vi "test_SessionReservationInfo_ReserveSessions_SessionAnnotationsPopulated.vi"(8 "error in":errorcluster) -> (0 "error out":errorcluster, 2 "result":string, 3 "pass":bool)   [LabVIEW 2021, in "MeasurementServerTests.lvlib" / "Session Reservation Tests.lvlib"]
uses:
  Session Reservation Tests.lvlib
  gRPC/Generated APIs/ni/measurementlink/sessionmanagement/v1/RPC Messages/ni_measurementlink_PinMapContext.ctl
  Runtime/Clients/Session Management V1/Session Reservation/Session Reservation.lvclass/Session Reservation.ctl
  bff49ccc-0781-4f8a-a739-0c4a6493da00.vi
  c21ecf1c-8bb5-4f68-90ba-61375d462941.vi
  Runtime/Clients/Session Management V1/Session Reservation/Merge Invalid DVR Error.vi
  Helpers/Pin Map XML Strings Global.vi
  Runtime/Clients/Session Management V1/Session Reservation/Is DVR Valid.vi
  Runtime/Measurements/Helpers/Error Strings Global Internal.vi
  <vilib>/Utility/error.llb/Error Cluster From Error Code.vi
  <vilib>/JDP Science/JSONtext/Variant to JSON Text.vi
  <vilib>/JDP Science/JSONtext/LVClass Serializer/JSONtext LVClass Serializer.lvclass
  gRPC/Generated APIs/ni/measurementlink/sessionmanagement/v1/ni.measurementlink.sessionmanagement.v1.api.lvlib
  MeasurementServerTests.lvlib
  Runtime/Clients/Session Management V1/Session Reservation/Session Reservation.lvclass
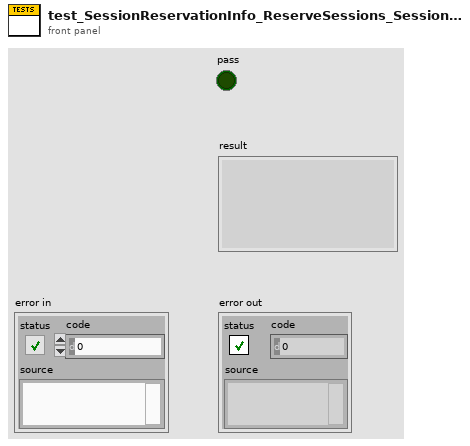
[diagram p1: front panel]
types:
  T1 = typedef "ni.measurementlink.sessionmanagement.v1.api.lvlib/ni_measurementlink_PinMapContext.ctl" = cluster{"pin_map_id":string, "sites":i32[]}
  T2 = typedef "ni.measurementlink.sessionmanagement.v1.api.lvlib/ni_measurementlink_sessionmanagement_v1_SessionInformation_AnnotationsEntry.ctl" = cluster{"key":string, "value":string}
  T3 = typedef "ni.measurementlink.sessionmanagement.v1.api.lvlib/ni_measurementlink_sessionmanagement_v1_SessionInformation.ctl" = cluster{"session":T4, "resource_name":string, "channel_list":string, "instrument_type_id":string, "session_exists":bool, "session_reserved":bool, "channel_mappings":T5[], "annotations":T2[]}
  T4 = typedef "ni.measurementlink.sessionmanagement.v1.api.lvlib/nidevice_grpc_Session.ctl" = cluster{"name":string}
  T5 = typedef "ni.measurementlink.sessionmanagement.v1.api.lvlib/ni_measurementlink_sessionmanagement_v1_ChannelMapping.ctl" = cluster{"pin_or_relay_name":string, "site":i32, "channel":string, "multiplexer_resource_name":string, "multiplexer_route":string}
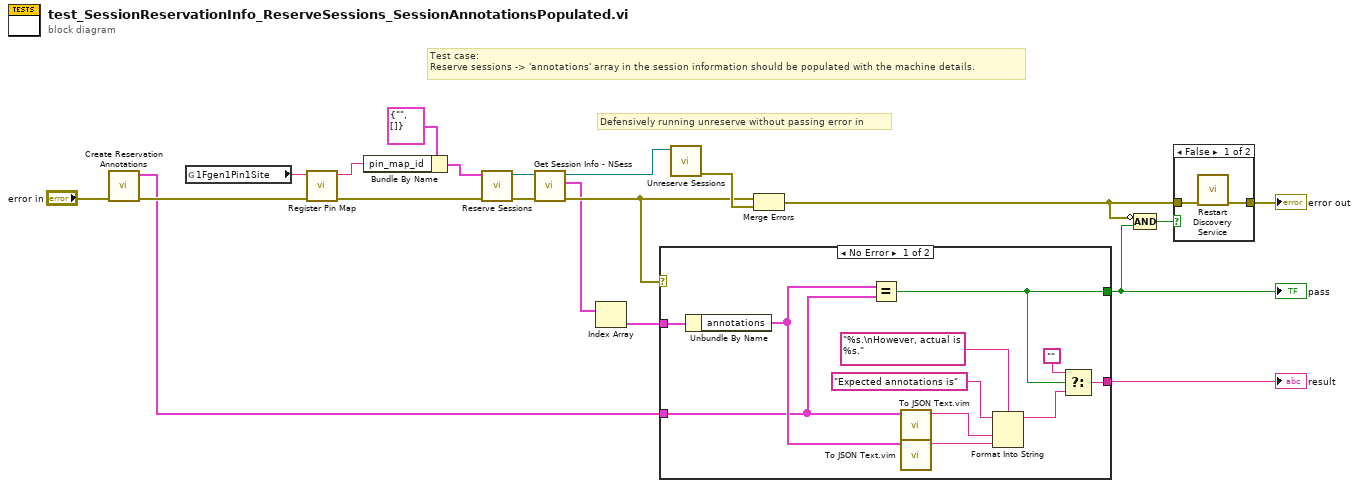
[diagram p0: block diagram]
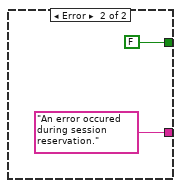
[diagram p3: hidden frame]
diagram:
  # "Defensively running unreserve without passing error in"
  # "Test case:\nReserve sessions -> 'annotations' array in the session information should be populated with the machine details."
  n1 = call "Create Reservation Annotations.vi"("error in"="error in") -> ("error out"=w10:errorcluster, "annotations array"=w6:T2[])  [unwired: 9 in]
  n2 = global read "Pin Map XML Strings Global.vi" "1Fgen1Pin1Site"() -> (w1:string)
  n3 = call "Register Pin Map.vi"("error in"=w10, "pin map xml"=w1) -> ("error out"=w16:errorcluster, "pin map id"=w17:string)  [unwired: 8 in]
  n4 = Bundle By Name(cluster=T1 {"pin_map_id"="", "sites"=[]} ("pin map context"), "pin_map_id"=w17) -> (w19:T1)
  n5 = call "Reserve Sessions.vi"("error in"=w16, "pin map context"=w19) -> ("error out"=w18:errorcluster, "session reservation out"=w5:refnum<class "Session Reservation.lvclass">)  [unwired: 8 in]
  n6 = call "Get Session Info - NSess .vi"("error in"=w18, "session reservation in"=w5) -> ("error out"=w9:errorcluster, "sessions info"=w7:T3[], "session reservation out"=w12:refnum<class "Session Reservation.lvclass">)  [unwired: 7 in]
  n7 = Index Array(array=w7) -> (element=w11:T3)  [unwired: 1 in]
  n8 = case shown="No Error" w9 {
    tunnel: [w22 FALSE] -> w4
    tunnel: [w27 "An error occured during session reservation." ("String")] -> w3
    tunnel: w11 -> [w23 _]
    tunnel: w6 -> [w21 _]
    frame No Error {
      n9 = Unbundle By Name(w23) -> ("annotations"=w25:T2[])
      n10 = Equal?(x=w25, y=w21) -> (x = y?=w22:bool)
      n11 = call "To JSON Text.vim"("Anything"=w21) -> ("<JSON>"=w24:string)  [unwired: 9 in, 1 out]
      n12 = call "To JSON Text.vim"("Anything"=w25) -> ("<JSON>"=w26:string)  [unwired: 9 in, 1 out]
      n13 = Format Into String(format string="%s.\nHowever, actual is %s.", initial string="Expected annotations is", w24, w26) -> (resulting string=w30:string)  [unwired: 1 in, 1 out]
      n14 = Select(t="", s=w22, f=w30) -> (s? t:f=w27:string)
    }
    frame Error {
    }
  }
  "pass" <- w4
  "result" <- w3
  n15 = call "Unreserve Sessions.vi"("session reservation in"=w12) -> ("error out"=w13:errorcluster)  [unwired: 10 in]
  n16 = Merge Errors(w9, w13) -> (w14:errorcluster)
  n17 = Compound Arithmetic op=AND(invert w14, w4) -> (w15:bool)
  n18 = case shown="False" w15 {
    tunnel: [w35 w36] -> w8
    tunnel: w14 -> [w34 w36]
    frame False {
      n19 = call "Restart Discovery Service.vi"("error in"=w34) -> ("error out"=w35:errorcluster)  [unwired: 10 in]
    }
    frame True {
    }
  }
  "error out" <- w8
